vi "MakeImagCondFileContents.vi"(9 "Cluster":T1, 10 "Position":string, 11 "StorageDirPath":path) -> (3 "StringOutToFile":string)   [LabVIEW 2016]
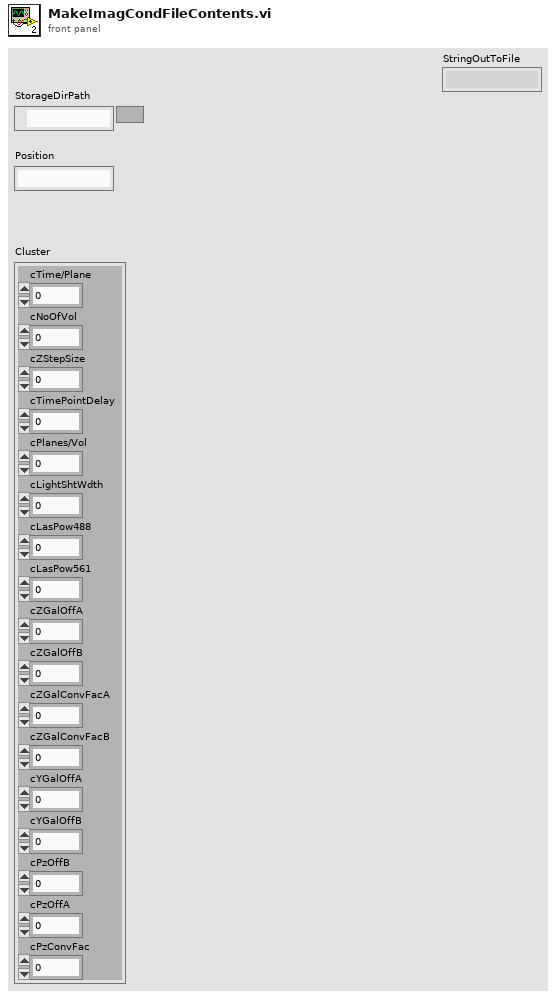
[diagram p1: front panel]
types:
  T1 = cluster{"cTime/Plane":dbl, "cNoOfVol":dbl, "cZStepSize":dbl, "cTimePointDelay":dbl, "cPlanes/Vol":dbl, "cLightShtWdth":dbl, "cLasPow488":dbl, "cLasPow561":dbl, "cZGalOffA":dbl, "cZGalOffB":dbl, "cZGalConvFacA":dbl, "cZGalConvFacB":dbl, "cYGalOffA":dbl, "cYGalOffB":dbl, "cPzOffB":dbl, "cPzOffA":dbl, "cPzConvFac":dbl}
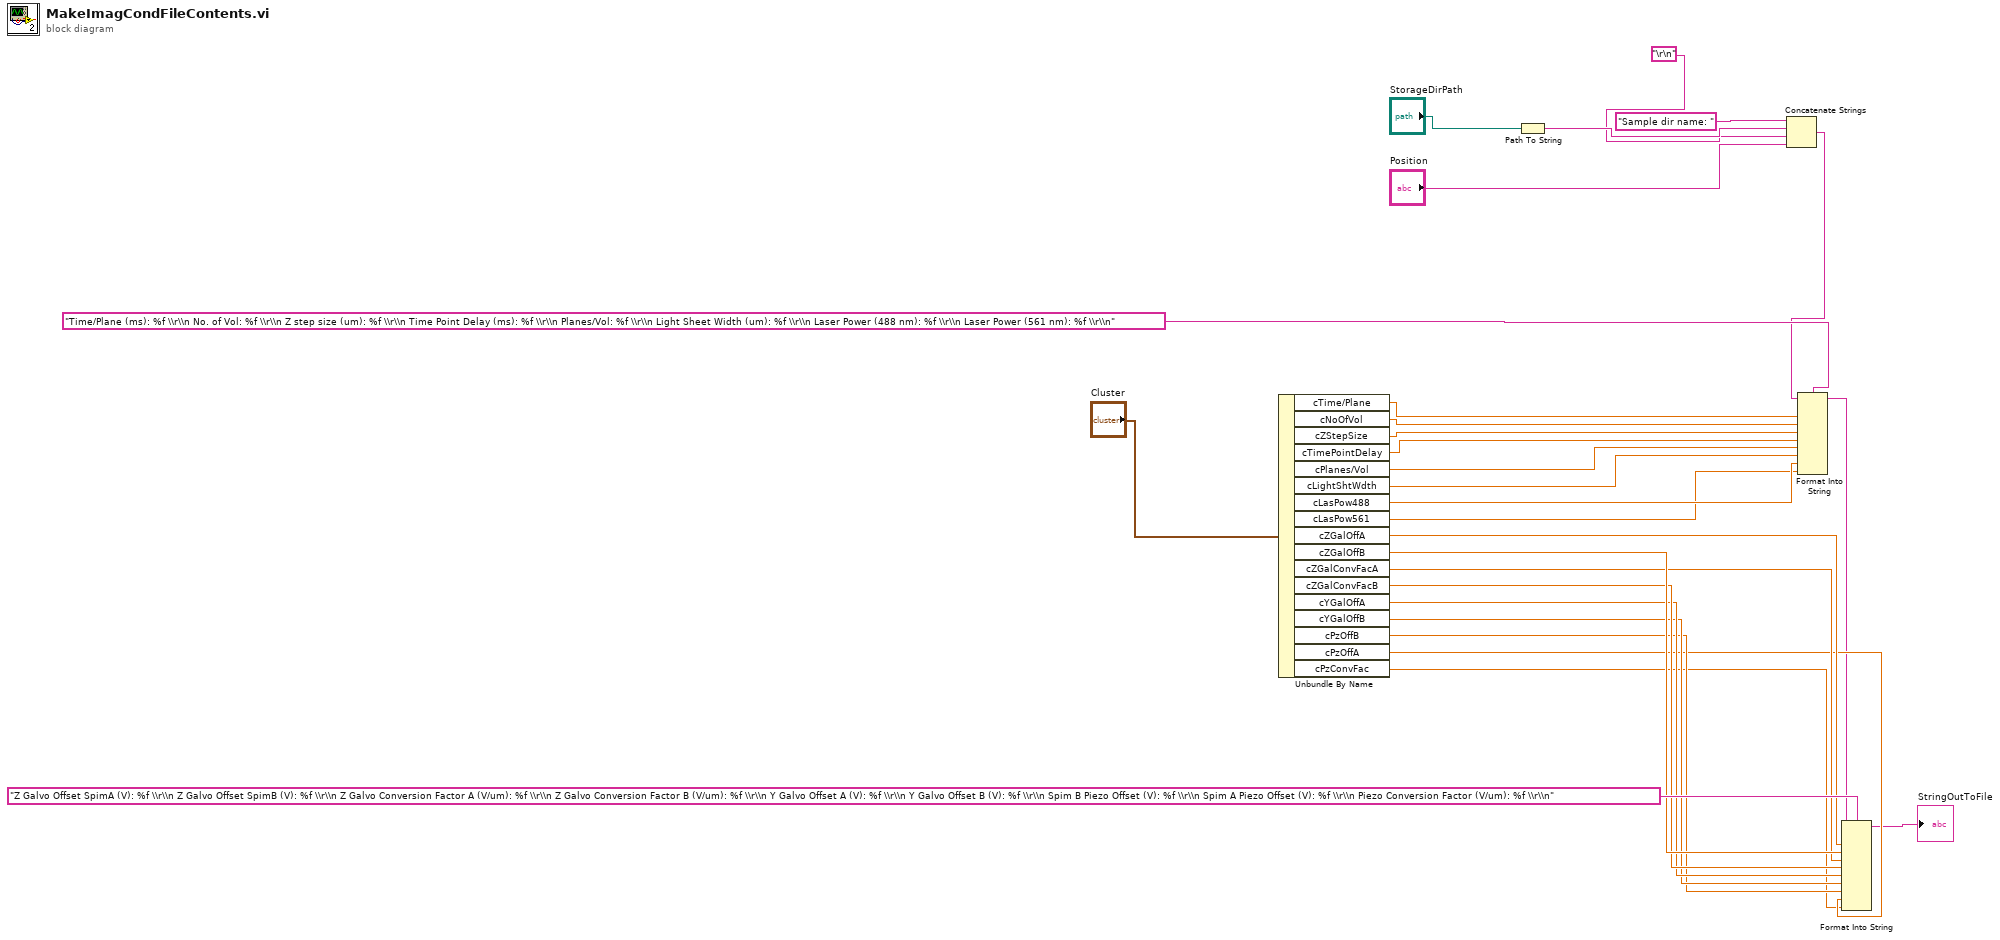
[diagram p0: block diagram]
diagram:
  n1 = Unbundle By Name("Cluster") -> ("cTime/Plane"=w22:dbl, "cNoOfVol"=w21:dbl, "cZStepSize"=w20:dbl, "cTimePointDelay"=w19:dbl, "cPlanes/Vol"=w18:dbl, "cLightShtWdth"=w17:dbl, "cLasPow488"=w16:dbl, "cLasPow561"=w15:dbl, "cZGalOffA"=w11:dbl, "cZGalOffB"=w10:dbl, "cZGalConvFacA"=w9:dbl, "cZGalConvFacB"=w8:dbl, "cYGalOffA"=w7:dbl, "cYGalOffB"=w6:dbl, "cPzOffB"=w5:dbl, "cPzOffA"=w4:dbl, "cPzConvFac"=w3:dbl)
  n2 = Path To String(path="StorageDirPath") -> (string=w26:string)
  n3 = Concatenate Strings("Sample dir name: " ("string"), w26, "\r\n", "Position") -> (w13:string)
  n4 = Format Into String(format string="Time/Plane (ms): %f \\r\\n No. of Vol: %f \\r\\n Z step size (um): %f \\r\\n Time Point Delay (ms): %f \\r\\n Planes/Vol: %f \\r\\n Light Sheet Width (um): %f \\r\\n Laser Power (488 nm): %f \\r\\n Laser Power (561 nm): %f \\r\\n" ("initial string"), initial string=w13, w22, w21, w20, w19, w18, w17, w16, w15) -> (resulting string=w2:string)  [unwired: 1 in, 1 out]
  n5 = Format Into String(format string="Z Galvo Offset SpimA (V): %f \\r\\n Z Galvo Offset SpimB (V): %f \\r\\n Z Galvo Conversion Factor A (V/um): %f \\r\\n Z Galvo Conversion Factor B (V/um): %f \\r\\n Y Galvo Offset A (V): %f \\r\\n Y Galvo Offset B (V): %f \\r\\n Spim B Piezo Offset (V): %f \\r\\n Spim A Piezo Offset (V): %f \\r\\n Piezo Conversion Factor (V/um): %f \\r\\n" ("initial string"), initial string=w2, w11, w10, w9, w8, w7, w6, w5, w4, w3) -> (resulting string=→"StringOutToFile":string)  [unwired: 1 in, 1 out]
